vi "From Serial Form.vi"(6 "Serial Version":T1, 10 "Deserializer in":refnum<class "Deserializer.lvclass">, 11 "String Data in":refnum<class "String Data.lvclass">) -> (0 "error out":errorcluster, 2 "Deserializer out":refnum<class "Deserializer.lvclass">, 3 "String Data out":refnum<class "String Data.lvclass">)   [LabVIEW 2014, in "Base Data Class.lvlib" / "String Data.lvclass"]
uses:
  String Data.lvclass
  <vilib>/NI/AQ Character Lineator/Deserializer/Deserializer.lvclass
  <vilib>/NI/AQ Character Lineator/Serialization Common/Serial Version.ctl
  String Data.lvclass/String Data.ctl
  <vilib>/NI/AQ Character Lineator/Serializable/Remove String.vi
  Data.lvclass
  <vilib>/NI/AQ Character Lineator/Serializable/Serializable.lvclass
  <vilib>/NI/AQ Character Lineator/Serialization Common/Serialization Common.lvlib
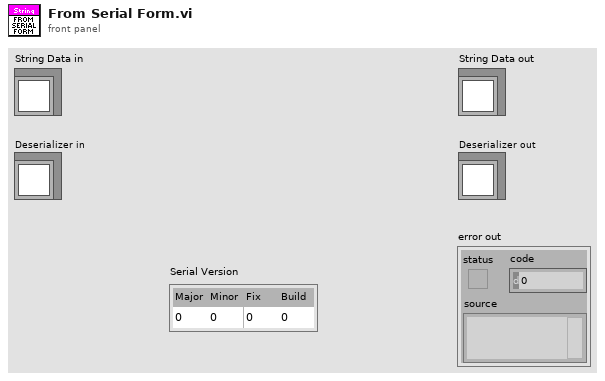
[diagram p1: front panel]
types:
  T1 = typedef "Serialization Common.lvlib/Serial Version.ctl" = cluster{"Major":u16, "Minor":u16, "Fix":u16, "Build":u16}
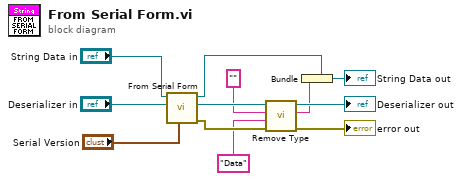
[diagram p0: block diagram]
diagram:
  n1 = call-parent "From Serial Form.vi"("Serial Version"="Serial Version", "Deserializer in"="Deserializer in", "Data in"="String Data in") -> ("error out"=w6:errorcluster, "Deserializer out"=w9:refnum<class "Deserializer.lvclass">, "Data out"=w3:refnum<class "String Data.lvclass">)  [unwired: 6 in]
  n2 = call-poly <vilib>:"Remove Type.vi"("error in (no error)"=w6, "Name"="Data", "Default Value"="", "Deserializer in"=w9) -> ("error out"=→"error out":errorcluster, "String"=w2:string, "Deserializer out"=→"Deserializer out":refnum<class "Deserializer.lvclass">)  [unwired: 4 in, 1 out]
  n3 = Bundle(cluster=w3, w2) -> (→"String Data out":refnum<class "String Data.lvclass">)
